vi "Main.vi"(11 "Module Admin":refnum<class "Delacor_lib_QMH_Cloneable Module Admin.lvclass">) -> ()   [LabVIEW 2019, in "Menu Module.lvlib"]
doc: "This template is based off of the Queued Message Handler design pattern and the Queued Message Handler project template that ships with LabVIEW.\n\nThe main difference is that the queue is private to this module and communication between modules is performed via Broadcast and Request events.\n\nRequest events are wrapped in public API methods and are handled in the Event Handling Loop (EHL) of this VI. Any module can register for Broadcast events sent by this module. The EHL generates messages based on user interface actions.\n\nThe Message Handling Loop (MHL) processes messages generated by the EHL, or by other messages. The messages are string values, so new messages can be added easily to the Message Cases case structure in the MHL. Each message cluster can also provide an optional value for Message Data, which is a variant that can be converted to whatever message-specific data is required.\n_____\nBased on Delacor QMH Project Template 5.0.0.82."
uses:
  Menu Module.lvlib
  <vilib>/Delacor/Delacor QMH/Libraries/Cloneable Module Admin_class/Delacor_lib_QMH_Cloneable Module Admin.lvclass
  C:/Program Files (x86)/National Instruments/LabVIEW 2019/vi.lib/Delacor/Delacor QMH/Libraries/Module Admin_class/Delacor_lib_QMH_Module Admin.lvclass
  Utility/Controls/Menu_Configuration.ctl
  Module Data--cluster.ctl
  <vilib>/Delacor/Delacor QMH/Libraries/Message Queue_class/Delacor_lib_QMH_Message Queue.lvclass/Delacor_lib_QMH_Message Queue.ctl
  <vilib>/Delacor/Delacor QMH/Libraries/Cloneable Module Admin_class/Delacor_lib_QMH_Cloneable Module Admin.lvclass/Delacor_lib_QMH_Cloneable Module Admin.ctl
  Stop Argument--cluster.ctl
  <vilib>/Delacor/Delacor QMH/Libraries/Module Admin_class/Delacor_lib_QMH_Module Admin.lvclass/Delacor_lib_QMH_Module Admin.ctl
  Init Menu Argument--cluster.ctl
  Resize the Panel Argument--cluster.ctl
  <vilib>/Utility/miscctls.llb/LVPointTypeDef.ctl
  <vilib>/Utility/miscctls.llb/LVRectTypeDef.ctl
  <vilib>/Delacor/Delacor QMH/Libraries/Message Queue_class/Delacor_lib_QMH_Enqueue Message (Single).vi
  <vilib>/Delacor/Delacor QMH/Libraries/Cloneable Module Admin_class/Delacor_lib_QMH_Get Module ID.vi
  <vilib>/Delacor/Delacor QMH/Libraries/Module Admin_class/Delacor_lib_QMH_Get External Launch.vi
  <vilib>/Utility/error.llb/Error Cluster From Error Code.vi
  <vilib>/ErrorRing/Error Ring.xnode
  <vilib>/Delacor/Delacor QMH/Libraries/Message Queue_class/Delacor_lib_QMH_Message Queue.lvclass
panel:
  in  "Select Module":i32(ring)=-1 caption="Select Module\nTo send Request to" items=["All"=-1]
  in  "Menu":T1(array[cluster])
  in  "Simulate MHL Error":bool
  in  "Simulate EHL Error":bool
  out "error out":errorcluster
  out "Status":string
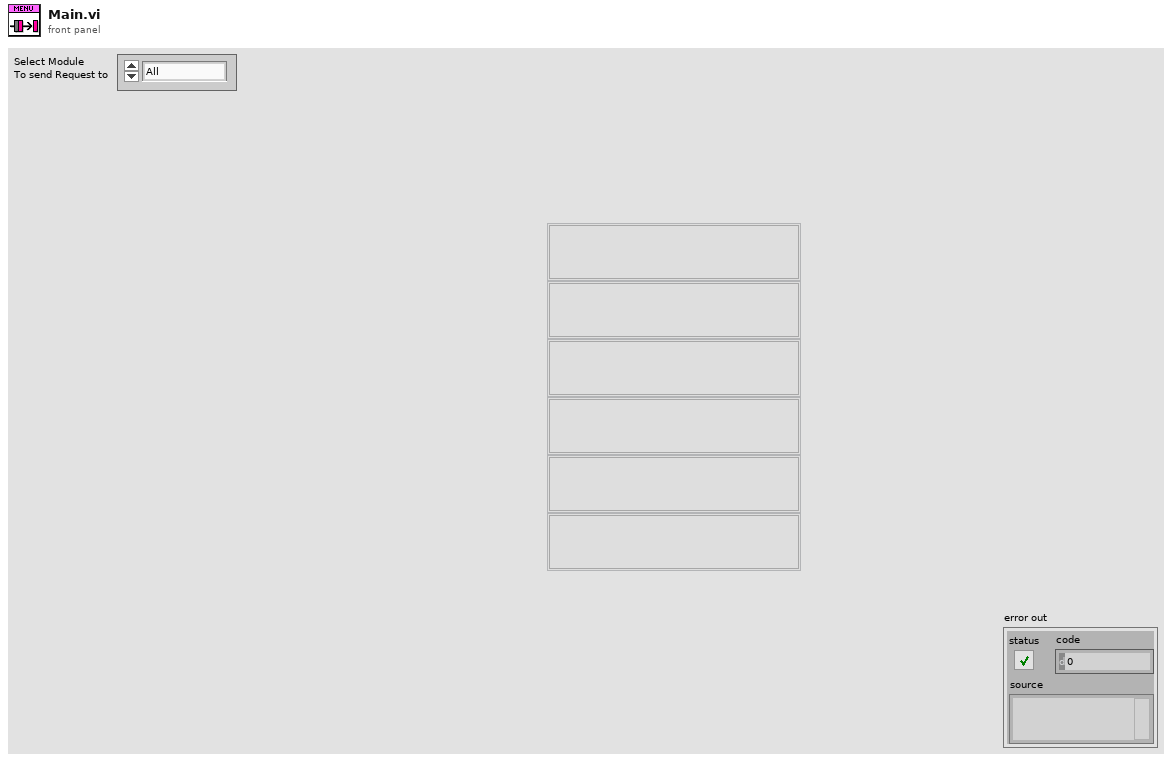
[diagram p1: front panel]
types:
  T1 = cluster{"Text ":string, "Icon":picture, "Button":bool, "Sub Menu":picture}[]
  T2 = typedef "Menu_Configuration.ctl" = cluster{"Button_Label_Color":u32, "Button_Color_On":u32, "Button_Color_Off":u32, "Panel_Color":u32, "Extend_Sub_Menu_Icon":path, "Root_Menu_Data":cluster{"Button_Icon":path, "Button_Label":string, "Sub_Menu_Data":cluster{"Button_Icon":path, "Button_Label":string, "Child_Menu_Data":cluster{"Button_Icon":path, "Button_Label":string}[]}[]}[]}
  T3 = cluster{"Text":string, "Menu_Configuration":T2, "Menu Type":enum16{"Root", "Sub", "Child"}, "Position":cluster{"Top":i16, "Left":i16}}
  T4 = typedef "Menu Module.lvlib/Request Events--cluster.ctl" = cluster{"Stop Module":refnum<user-event>, "Show Panel":refnum<user-event>, "Hide Panel":refnum<user-event>, "Show Diagram":refnum<user-event>, "Get Module Execution Status":refnum<user-event>, "Init Menu":refnum<user-event>, "Resize the Panel":refnum<user-event>}
  T5 = typedef "Menu Module.lvlib/Broadcast Events--cluster.ctl" = cluster{"Module Did Init":refnum<user-event>, "Status Updated":refnum<user-event>, "Error Reported":refnum<user-event>, "Module Did Stop":refnum<user-event>, "Update Module Execution Status":refnum<user-event>, "Button Pressed":refnum<user-event>}
  T6 = typedef "Menu Module.lvlib/Module Data--cluster.ctl" = cluster{"Status":string, "Menu_Configuration":T2, "Menu Type":enum16{"Root", "Sub", "Child"}, "Parent Name":string}
  T7 = enum32{"invalid lock state", "Not Locked", "Locked (No Password)", "Password-protected"}
  T8 = typedef "Menu Module.lvlib/Stop Argument--cluster.ctl" = cluster{"Module ID":i32, "Origin":string, "Exit via Stop Module Req?":bool, "Wait for Module to stop?":bool}
  T9 = typedef "Menu Module.lvlib/Init Menu Argument--cluster.ctl" = cluster{"Module ID":i32, "Menu_Configuration":T2, "Menu Type":enum16{"Root", "Sub", "Child"}, "Parent Name":string}
  T10 = typedef "Menu Module.lvlib/Resize the Panel Argument--cluster.ctl" = cluster{"Module ID":i32, "Boolean":bool, "Position":cluster{"Top":i16, "Left":i16}}
  T11 = typedef "LVPointTypeDef.ctl" = cluster{"Horizontal":i16, "Vertical":i16}
  T12 = enum32{"Invalid", "Standard", "Closed", "Hidden", "Minimized", "Maximized"}
  T13 = typedef "LVRectTypeDef.ctl" = cluster{"Left":i16, "Top":i16, "Right":i16, "Bottom":i16}
  T14 = typedef "LVPoint32TypeDef.ctl" = cluster{"Horizontal":i32, "Vertical":i32}
  T15 = typedef "LVPositionTypeDef.ctl" = cluster{"Left":i32, "Top":i32}
  T16 = cluster{"Text ":string, "Icon":picture, "Button":bool, "Sub Menu":picture}
  T17 = typedef "LVBoundsTypeDef.ctl" = cluster{"Width":u32, "Height":u32}
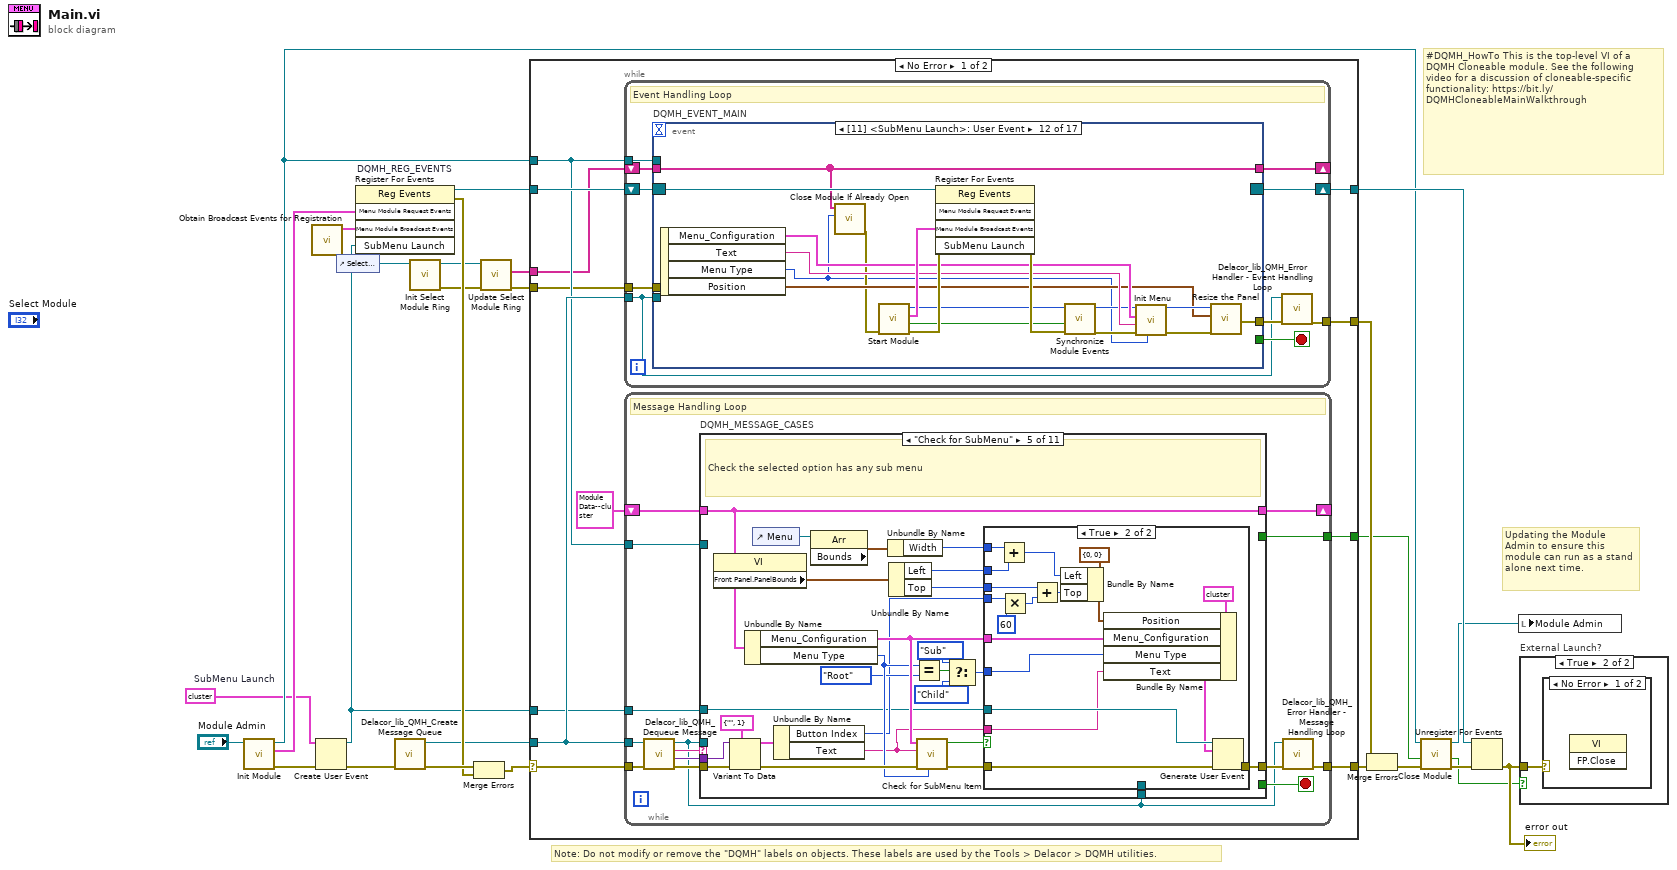
[diagram p0: block diagram]
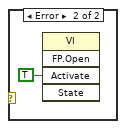
[diagram p3: hidden frame]
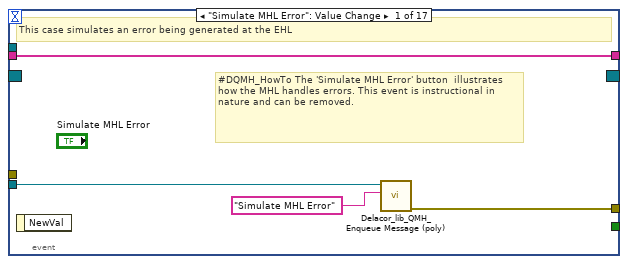
[diagram p4: hidden frame]
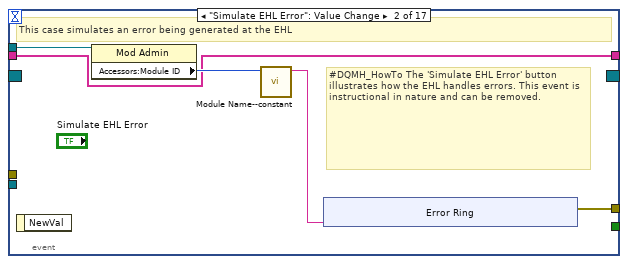
[diagram p5: hidden frame]
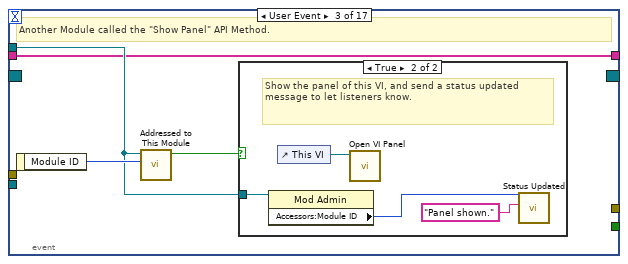
[diagram p6: hidden frame]
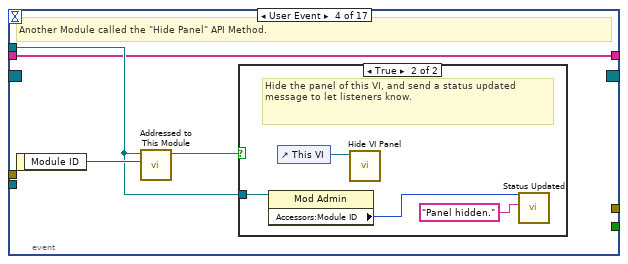
[diagram p8: hidden frame]
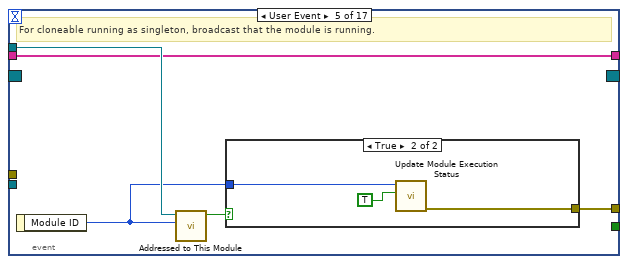
[diagram p10: hidden frame]
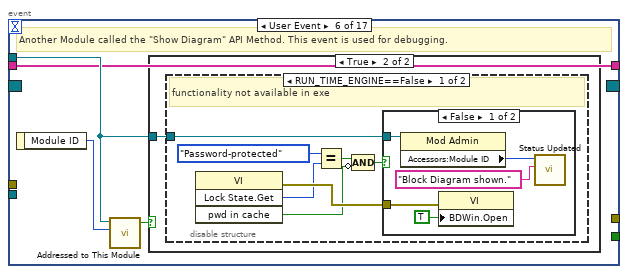
[diagram p12: hidden frame]
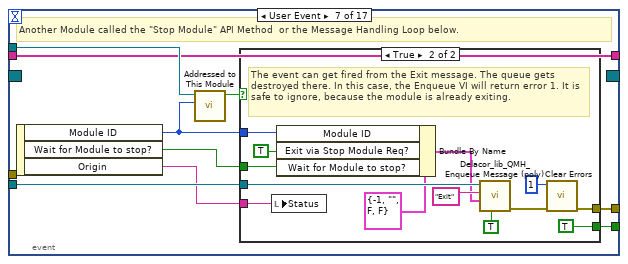
[diagram p16: hidden frame]
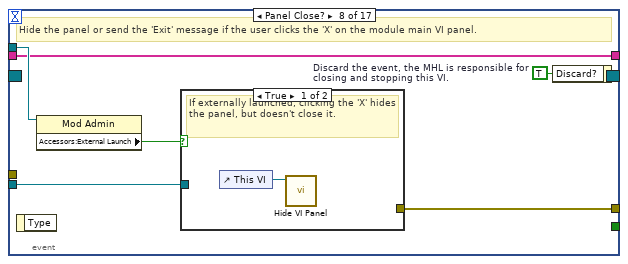
[diagram p18: hidden frame]
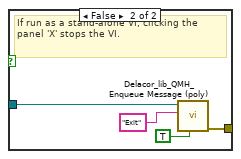
[diagram p19: hidden frame]
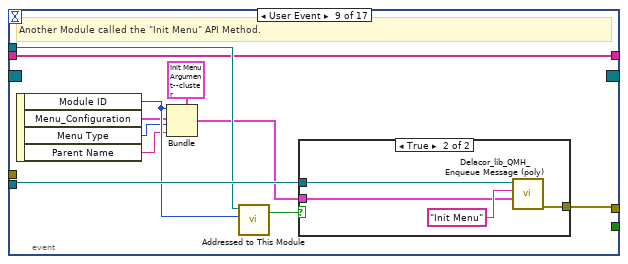
[diagram p20: hidden frame]
diagram:
  w6 = T3 {"Text"="", "Menu_Configuration"={"Button_Label_Color"=2344, "Button_Color_On"=5654, "Button_Color_Off"=2344, "Panel_Color"=2344, "Extend_Sub_Menu_Icon"=path "C:/Users/SyncSols-4/Desktop/Icon/Accept-icon.png", "Root_Menu_Data"=[{"Button_Icon"=path "C:/Users/SyncSols-4/Desktop/Icon/Accept-icon.png", "Button_Label"="Test", "Sub_Menu_Data"=[{"Button_Icon"=path "C:/Users/SyncSols-4/Desktop/Icon/floppy-icon.png", "Button_Label"="Save", "Child_Menu_Data"=[]}, {"Button_Icon"=path "C:/Users/SyncSols-4/Desktop/Icon/folder-icon1.png", "Button_Label"="Folder", "Child_Menu_Data"=[]}, {"Button_Icon"=path "C:/Users/SyncSols-4/Desktop/Icon/delete-icon.png", "Button_Label"="Delete", "Child_Menu_Data"=[{"Button_Icon"=path "C:/Users/SyncSols-4/Desktop/Icon/add-icon.png", "Button_Label"="Add"}, {"Button_Icon"=path "C:/Users/SyncSols-4/Desktop/Icon/Stop-red-icon.png", "Button_Label"="Stop"}]}]}, {"Button_Icon"=path "C:/Users/SyncSols-4/Desktop/Icon/add-key-icon.png", "Button_Label"="Key", "Sub_Menu_Data"=[]}, {"Button_Icon"=path "C:/Users/SyncSols-4/Desktop/Icon/Categories-preferences-system-icon.png", "Button_Label"="Setting", "Sub_Menu_Data"=[]}]}, "Menu Type"=enum."Root", "Position"={"Top"=0, "Left"=0}}  # SubMenu Launch
  # "#DQMH_HowTo This is the top-level VI of a DQMH Cloneable module. See the following video for a discussion of cloneable-specific functionality: https://bit.ly/DQMHCloneableMainWalkthrough"
  # "Note: Do not modify or remove the \"DQMH\" labels on objects. These labels are used by the Tools > Delacor > DQMH utilities."
  # "Updating the Module Admin to ensure this module can run as a stand alone next time."
  n1 = call "Init Module.vi"("Cloneable Module Admin in"="Module Admin") -> ("error out"=w8:errorcluster, "Menu Module Request Events"=w17:T4, "Cloneable Module Admin out"=w14:refnum<class "Delacor_lib_QMH_Cloneable Module Admin.lvclass">)  [unwired: 8 in]
  n2 = call "Obtain Broadcast Events for Registration.vi"() -> ("Menu Module Broadcast Events"=w10:T5)  [unwired: 9 in, 2 out]
  n3 = Create User Event(user event datatype=w6, error in=w8) -> (user event=w5:refnum<user-event>, error out=w7:errorcluster)
  n4 = control-ref of="Select Module"() -> (w2:refnum<vi>)
  n5 = register-events "DQMH_REG_EVENTS"(w17, w10, w5) -> (reference out=w9:refnum<event-registration>, error out=w19:errorcluster)  [unwired: 2 in]
  n6 = call <vilib>:"Delacor_lib_QMH_Create Message Queue.vi"("error in"=w7) -> ("error out"=w21:errorcluster, "Message Queue"=w16:refnum<class "Delacor_lib_QMH_Message Queue.lvclass">)  [unwired: 9 in]
  n7 = call "Init Select Module Ring.vi"("Select Module Ring Ref"=w2) -> ("error out"=w4:errorcluster)  [unwired: 8 in, 2 out]
  n8 = Merge Errors(w21, w19) -> (w20:errorcluster)
  n9 = call "Update Select Module Ring.vi"("error in (no error)"=w4, "Select Module Ring Ref"=w2) -> ("error out"=w3:errorcluster, "Active Modules (Array)"=w1:string[])  [unwired: 7 in, 1 out]
  n10 = case shown="No Error" w20 {
    selector: w20 -> [w36 w440]
    tunnel: [w38 w439] -> w24
    tunnel: [w35 w447] -> w18
    tunnel: w9 -> [w33 w447]
    tunnel: w16 -> [w32 w438]
    tunnel: [w37 _] -> w25
    tunnel: w14 -> [w31 w443]
    tunnel: [w30 _] -> w12
    tunnel: w5 -> [w29 _]
    tunnel: w3 -> [w28 _]
    tunnel: w1 -> [w27 _]
    frame No Error {
      n11 = while {
        tunnel: w32 -> [w42]
        shift-right: [w45] -> w35
        shift-left: w33 -> [w46]
        tunnel: [w47] -> w37
        tunnel: w31 -> [w43]
        shift-right: [w41] -> _
        shift-left: w27 -> [w40]
        tunnel: w28 -> [w39]
        stop <- w44 stop-if-true
        # "Event Handling Loop"
        n12 = event "DQMH_EVENT_MAIN" shown="[11] <SubMenu Launch>: User Event" {
          selector: w46 -> [_ _ _ _ _ _ _ _ _ _ _ w195 _ w209 w213 _ _]
          dyn-events: [_ _ _ _ _ _ _ _ _ _ _ _ _ w207 w213 _ _] -> w45
          timeout: _ -> [_ _ _ _ _ _ _ _ _ _ _ _ _ _ _ _ _]
          tunnel: [_ _ _ _ _ _ w110 _ _ _ _ _ _ _ _ _ _] -> w44
          tunnel: w42 -> [w51 _ _ _ _ _ w113 w130 w149 w163 w174 _ w202 _ _ w225 _]
          tunnel: [w52 w57 _ _ w85 _ w114 w133 w142 w156 w175 w183 w203 w206 w210 w224 w238] -> w48
          tunnel: w43 -> [_ w56 w66 w74 w83 w90 w112 w131 w147 w161 _ _ w201 _ _ w223 w237]
          tunnel: [w49 w53 w65 w73 w81 w89 w106 w128 w139 w154 w168 w181 w200 w205 w212 w219 w233] -> w41
          tunnel: w40 -> [w49 w53 w65 w73 w81 w89 w106 w128 w139 w154 w168 w181 w200 _ _ w219 w233]
          tunnel: w39 -> [_ _ _ _ _ _ _ _ _ _ _ _ _ _ _ _ _]
          event "Simulate MHL Error": Value Change {
            # "#DQMH_HowTo The 'Simulate MHL Error' button  illustrates how the MHL handles errors. This event is instructional in nature and can be removed."
            # "This case simulates an error being generated at the EHL"
            n13 = event-data() -> ()  [unwired: 1 in, 1 out]
            n14 = call-poly <vilib>:"Delacor_lib_QMH_Enqueue Message (poly).vi"("Message"="Simulate MHL Error", "Message Queue in"=w51) -> ("error out"=w52:errorcluster)  [unwired: 8 in, 1 out]
          }
          event "Simulate EHL Error": Value Change {
            # "#DQMH_HowTo The 'Simulate EHL Error' button  illustrates how the EHL handles errors. This event is instructional in nature and can be removed."
            # "This case simulates an error being generated at the EHL"
            n15 = event-data() -> ()  [unwired: 1 in, 1 out]
            n16 = property class="Mod Admin"(reference=w56) -> ("Accessors:Module ID"=w55:i32)  [unwired: 1 in, 2 out]
            n17 = call "Module Name--constant.vi"("Module ID"=w55) -> ("Module Name"=w54:string)  [unwired: 10 in]
            n18 = xnode "Error Ring"("parameter 0"=w54) -> ("error out"=w57:errorcluster)
          }
          event User Event {
            # "Another Module called the \"Show Panel\" API Method."
            n19 = event-data() -> ("Module ID"=w67:i32)  [unwired: 1 in]
            n20 = call "Addressed to This Module.vi"("Module ID from Argument"=w67, "Module Admin"=w66) -> ("Addressed to this instance?"=w68:bool)  [unwired: 8 in, 1 out]
            n21 = case shown="True" w68 {
              tunnel: w66 -> [_ w70]
              frame False {
              }
              frame True {
                # "Show the panel of this VI, and send a status updated message to let listeners know."
                n22 = property class="Mod Admin"(reference=w70) -> ("Accessors:Module ID"=w69:i32)  [unwired: 1 in, 2 out]
                n23 = control-ref of="This VI"() -> (w72:refnum<vi>)
                n24 = call "Open VI Panel.vi"("VI"=w72) -> ()  [unwired: 10 in, 1 out]
                n25 = call "Status Updated.vi"("Status"="Panel shown." ("format string"), "Module ID"=w69) -> ()  [unwired: 9 in, 1 out]
              }
            }
          }
          event User Event {
            # "Another Module called the \"Hide Panel\" API Method."
            n26 = event-data() -> ("Module ID"=w75:i32)  [unwired: 1 in]
            n27 = call "Addressed to This Module.vi"("Module ID from Argument"=w75, "Module Admin"=w74) -> ("Addressed to this instance?"=w76:bool)  [unwired: 8 in, 1 out]
            n28 = case shown="True" w76 {
              tunnel: w74 -> [_ w78]
              frame False {
              }
              frame True {
                # "Hide the panel of this VI, and send a status updated message to let listeners know."
                n29 = property class="Mod Admin"(reference=w78) -> ("Accessors:Module ID"=w77:i32)  [unwired: 1 in, 2 out]
                n30 = control-ref of="This VI"() -> (w80:refnum<vi>)
                n31 = call "Hide VI Panel.vi"("VI"=w80) -> ()  [unwired: 10 in, 1 out]
                n32 = call "Status Updated.vi"("Status"="Panel hidden." ("format string"), "Module ID"=w77) -> ()  [unwired: 9 in, 1 out]
              }
            }
          }
          event User Event {
            # "For cloneable running as singleton, broadcast that the module is running."
            n33 = event-data() -> ("Module ID"=w82:i32)  [unwired: 1 in]
            n34 = call "Addressed to This Module.vi"("Module ID from Argument"=w82, "Module Admin"=w83) -> ("Addressed to this instance?"=w84:bool)  [unwired: 8 in, 1 out]
            n35 = case shown="True" w84 {
              tunnel: [_ w88] -> w85
              tunnel: w82 -> [_ w87]
              frame False {
              }
              frame True {
                n36 = call "Update Module Execution Status.vi"("Running?"=TRUE, "Module ID"=w87) -> ("error out"=w88:errorcluster)  [unwired: 9 in]
              }
            }
          }
          event User Event {
            # "Another Module called the \"Show Diagram\" API Method. This event is used for debugging."
            n37 = event-data() -> ("Module ID"=w91:i32)  [unwired: 1 in]
            n38 = call "Addressed to This Module.vi"("Module ID from Argument"=w91, "Module Admin"=w90) -> ("Addressed to this instance?"=w92:bool)  [unwired: 8 in, 1 out]
            n39 = case shown="True" w92 {
              tunnel: w90 -> [_ w93]
              frame False {
              }
              frame True {
                n40 = disable-structure shown="RUN_TIME_ENGINE==False" {
                  disable-tunnel: w93 -> [w94 _]
                  frame condition #0 (active) {
                    # "functionality not available in exe"
                    n41 = invoke class="VI" method="Lock State.Get"() -> (error out=w100:errorcluster, "Get Lock State"=w99:T7, "pwd in cache"=w96:bool)  [unwired: 4 in, 1 out]
                    n42 = Equal?(x=T7."Password-protected", y=w99) -> (x = y?=w97:bool)
                    n43 = Compound Arithmetic op=AND(w97, invert w96) -> (w95:bool)
                    n44 = case shown="False" w95 {
                      tunnel: w100 -> [w105 _]
                      tunnel: w94 -> [w102 _]
                      frame False {
                        n45 = property class="Mod Admin"(reference=w102) -> ("Accessors:Module ID"=w101:i32)  [unwired: 1 in, 2 out]
                        n46 = property class="VI"(error in=w105, "BDWin.Open"=TRUE ("Block Diagram Window:Open")) -> ()  [unwired: 1 in, 2 out]
                        n47 = call "Status Updated.vi"("Status"="Block Diagram shown." ("format string"), "Module ID"=w101) -> ()  [unwired: 9 in, 1 out]
                      }
                      frame True {
                        # "Password-protected VI, and the password is not in the cache. Do not show the diagram."
                      }
                    }
                  }
                  frame condition #1 {
                  }
                }
              }
            }
          }
          event User Event {
            # "Another Module called the \"Stop Module\" API Method  or the Message Handling Loop below."
            n48 = event-data() -> ("Module ID"=w108:i32, "Wait for Module to stop?"=w109:bool, "Origin"=w107:string)  [unwired: 1 in]
            n49 = call "Addressed to This Module.vi"("Module ID from Argument"=w108, "Module Admin"=w112) -> ("Addressed to this instance?"=w111:bool)  [unwired: 8 in, 1 out]
            n50 = case shown="True" w111 {
              tunnel: [_ w126] -> w114
              tunnel: w113 -> [_ w122]
              tunnel: [_ TRUE] -> w110
              tunnel: w109 -> [_ w117]
              tunnel: w108 -> [_ w119]
              tunnel: w107 -> [_ w115]
              frame False {
              }
              frame True {
                # "The event can get fired from the Exit message. The queue gets destroyed there. In this case, the Enqueue VI will return error 1. It is safe to ignore, because the module is already exiting."
                n51 = local write "Status"(w115) -> ()
                n52 = Bundle By Name(cluster=T8 {"Module ID"=-1, "Origin"="", "Exit via Stop Module Req?"=FALSE, "Wait for Module to stop?"=FALSE} ("Stop Argument"), "Module ID"=w119, "Exit via Stop Module Req?"=TRUE, "Wait for Module to stop?"=w117) -> (w116:T8)
                n53 = call-poly <vilib>:"Delacor_lib_QMH_Enqueue Message (poly).vi"("Priority Message? (F)"=TRUE, "Message Data"=w116, "Message"="Exit", "Message Queue in"=w122) -> ("error out"=w127:errorcluster)  [unwired: 6 in, 1 out]
                n54 = call <vilib>:"Clear Errors.vi"("error in (no error)"=w127, "specific error code to clear (0: all)"=1) -> ("error out"=w126:errorcluster)  [unwired: 4 in, 1 out]
              }
            }
          }
          event Panel Close? {
            w132 = TRUE  # Discard the event, the MHL is responsible for closing and stopping this VI.
            # "Hide the panel or send the 'Exit' message if the user clicks the 'X' on the module main VI panel."
            n55 = event-data() -> ()  [unwired: 1 in, 1 out]
            n56 = property class="Mod Admin"(reference=w131) -> ("Accessors:External Launch"=w129:bool)  [unwired: 1 in, 2 out]
            n57 = case shown="True" w129 {
              tunnel: w130 -> [_ w137]
              tunnel: [_ w138] -> w133
              frame True {
                # "If externally launched, clicking the 'X' hides the panel, but doesn't close it."
                n58 = control-ref of="This VI"() -> (w134:refnum<vi>)
                n59 = call "Hide VI Panel.vi"("VI"=w134) -> ()  [unwired: 10 in, 1 out]
              }
              frame False {
                # "If run as a stand-alone VI, clicking the panel 'X' stops the VI."
                n60 = call-poly <vilib>:"Delacor_lib_QMH_Enqueue Message (poly).vi"("Priority Message? (F)"=TRUE, "Message"="Exit", "Message Queue in"=w137) -> ("error out"=w138:errorcluster)  [unwired: 7 in, 1 out]
              }
            }
            n61 = event-data("Discard?"=w132) -> ()  [unwired: 1 in, 1 out]
          }
          event User Event {
            # "Another Module called the \"Init Menu\" API Method."
            n62 = event-data() -> ("Module ID"=w144:i32, "Menu_Configuration"=w143:T2, "Menu Type"=w141:enum16{"Root", "Sub", "Child"}, "Parent Name"=w140:string)  [unwired: 1 in]
            n63 = Bundle(cluster=T9 {"Module ID"=-1, "Menu_Configuration"={"Button_Label_Color"=2344, "Button_Color_On"=5654, "Button_Color_Off"=2344, "Panel_Color"=2344, "Extend_Sub_Menu_Icon"=path "C:/Users/SyncSols-4/Desktop/Icon/Accept-icon.png", "Root_Menu_Data"=[{"Button_Icon"=path "C:/Users/SyncSols-4/Desktop/Icon/Accept-icon.png", "Button_Label"="Test", "Sub_Menu_Data"=[{"Button_Icon"=path "C:/Users/SyncSols-4/Desktop/Icon/floppy-icon.png", "Button_Label"="Save", "Child_Menu_Data"=[]}, {"Button_Icon"=path "C:/Users/SyncSols-4/Desktop/Icon/folder-icon1.png", "Button_Label"="Folder", "Child_Menu_Data"=[]}, {"Button_Icon"=path "C:/Users/SyncSols-4/Desktop/Icon/delete-icon.png", "Button_Label"="Delete", "Child_Menu_Data"=[{"Button_Icon"=path "C:/Users/SyncSols-4/Desktop/Icon/add-icon.png", "Button_Label"="Add"}, {"Button_Icon"=path "C:/Users/SyncSols-4/Desktop/Icon/Stop-red-icon.png", "Button_Label"="Stop"}]}]}, {"Button_Icon"=path "C:/Users/SyncSols-4/Desktop/Icon/add-key-icon.png", "Button_Label"="Key", "Sub_Menu_Data"=[]}, {"Button_Icon"=path "C:/Users/SyncSols-4/Desktop/Icon/Categories-preferences-system-icon.png", "Button_Label"="Setting", "Sub_Menu_Data"=[]}]}, "Menu Type"=enum."Root", "Parent Name"=""} ("Init Menu Argument"), "Module ID"=w144, "Menu_Configuration"=w143, "Menu Type"=w141, "Parent Name"=w140) -> (w145:T9)
            n64 = call "Addressed to This Module.vi"("Module ID from Argument"=w144, "Module Admin"=w147) -> ("Addressed to this instance?"=w148:bool)  [unwired: 8 in, 1 out]
            n65 = case shown="True" w148 {
              tunnel: w149 -> [_ w153]
              tunnel: w145 -> [_ w151]
              tunnel: [_ w150] -> w142
              frame False {
              }
              frame True {
                n66 = call-poly <vilib>:"Delacor_lib_QMH_Enqueue Message (poly).vi"("Message Data"=w151, "Message"="Init Menu", "Message Queue in"=w153) -> ("error out"=w150:errorcluster)  [unwired: 7 in, 1 out]
              }
            }
          }
          event User Event {
            # "Another Module called the \"Resize the Panel\" API Method."
            n67 = event-data() -> ("Module ID"=w158:i32, "Boolean"=w157:bool, "Position"=w155:cluster{"Top":i16, "Left":i16})  [unwired: 1 in]
            n68 = Bundle(cluster=T10 {"Module ID"=-1, "Boolean"=FALSE, "Position"={"Top"=100, "Left"=100}} ("Resize the Panel Argument"), "Module ID"=w158, "Boolean"=w157, "Position"=w155) -> (w159:T10)
            n69 = call "Addressed to This Module.vi"("Module ID from Argument"=w158, "Module Admin"=w161) -> ("Addressed to this instance?"=w162:bool)  [unwired: 8 in, 1 out]
            n70 = case shown="True" w162 {
              tunnel: w163 -> [_ w167]
              tunnel: w159 -> [_ w165]
              tunnel: [_ w164] -> w156
              frame False {
              }
              frame True {
                n71 = call-poly <vilib>:"Delacor_lib_QMH_Enqueue Message (poly).vi"("Message Data"=w165, "Message"="Resize the Panel", "Message Queue in"=w167) -> ("error out"=w164:errorcluster)  [unwired: 7 in, 1 out]
              }
            }
          }
          event "Menu": Mouse Down {
            n72 = event-data() -> ("Coords"=w179:T14)  [unwired: 1 in]
            n73 = property on="Menu" class="Arr"() -> ("Position"=w178:T15)  [unwired: 2 in, 2 out]
            n74 = call "Find Mouse Down Option.vi"("Menu Position"=w178, "Mouse DownCoords"=w179) -> ("Button Index"=w171:u32)  [unwired: 8 in, 1 out]
            n75 = Index Array(array="Menu", index=w171) -> (element=w176:T16)
            n76 = Unbundle By Name(w176) -> ("Text"=w172:string)
            n77 = Bundle By Name(cluster=cluster{"Text":string, "Button Index":u32} {"Text"="", "Button Index"=1}, "Text"=w172, "Button Index"=w171) -> (w170:cluster{"Text":string, "Button Index":u32})
            n78 = call-poly <vilib>:"Delacor_lib_QMH_Enqueue Message (poly).vi"("Message Data"=w170, "Message"="Check for SubMenu", "Message Queue in"=w174) -> ("error out"=w175:errorcluster)  [unwired: 7 in, 1 out]
          }
          event User Event {
            n79 = event-data() -> ("Menu_Configuration"=w188:T2, "Text"=w187:string, "Menu Type"=w180:enum16{"Root", "Sub", "Child"}, "Position"=w184:cluster{"Top":i16, "Left":i16})  [unwired: 1 in]
            n80 = call "Close Module If Already Open.vi"("Menu Type"=w180, "Module List"=w181) -> ("error out"=w182:errorcluster)  [unwired: 9 in]
            n81 = call "Start Module.vi"("error in (no error)"=w182) -> ("error out"=w193:errorcluster, "Wait for Event Sync?"=w190:bool, "Menu Module Broadcast Events"=w194:T5, "Module ID"=w191:i32)  [unwired: 7 in]
            n82 = register-events(reference=w195, error in=w193, w194) -> (error out=w192:errorcluster)  [unwired: 2 in, 1 out]
            n83 = call "Synchronize Module Events.vi"("error in (no error)"=w192, "Wait for Event Sync?"=w190, "Module ID"=w191) -> ("error out"=w189:errorcluster, "Module ID (dup)"=w186:i32)  [unwired: 7 in]
            n84 = call "Init Menu.vi"("Menu Type"=w180, "error in (no error)"=w189, "Parent Name"=w187, "Menu_Configuration"=w188, "Module ID"=w186) -> ("error out"=w185:errorcluster)  [unwired: 6 in]
            n85 = call "Resize the Panel.vi"("error in (no error)"=w185, "Position"=w184, "Module ID"=w186) -> ("error out"=w183:errorcluster)  [unwired: 8 in]
          }
          event User Event {
            n86 = event-data() -> ()  [unwired: 1 in, 1 out]
            n87 = property class="Mod Admin"(reference=w201) -> ("Accessors:Module ID"=w198:i32)  [unwired: 1 in, 2 out]
            n88 = Number To Decimal String(number=w198) -> (decimal integer string=w199:string)  [unwired: 1 in]
            n89 = Search 1D Array(1D array=w200, element=w199) -> (index of element=w197:i32)  [unwired: 1 in]
            n90 = Equal To 0?(x=w197) -> ()  [unwired: 1 out]
            n91 = call-poly <vilib>:"Delacor_lib_QMH_Enqueue Message (poly).vi"("Message"="Exit", "Message Queue in"=w202) -> ("error out"=w203:errorcluster)  [unwired: 8 in, 1 out]
          }
          event User Event {
            n92 = event-data() -> ()  [unwired: 1 in, 2 out]
            n93 = call "Obtain Broadcast Events for Registration.vi"() -> ("error out"=w206:errorcluster, "Menu Module Broadcast Events"=w208:T5)  [unwired: 9 in, 1 out]
            n94 = register-events "Reg Event"(reference=w209, w208) -> (reference out=w207:refnum<event-registration>)  [unwired: 3 in, 1 out]
            n95 = control-ref of="Select Module"() -> (w204:refnum<vi>)
            n96 = call "Update Select Module Ring.vi"("error in (no error)"=w206, "Select Module Ring Ref"=w204) -> ("Active Modules (Array)"=w205:string[])  [unwired: 7 in, 2 out]
          }
          event User Event {
            n97 = event-data() -> ()  [unwired: 1 in, 2 out]
            n98 = control-ref of="Select Module"() -> (w211:refnum<vi>)
            n99 = call "Update Select Module Ring.vi"("Select Module Ring Ref"=w211) -> ("error out"=w210:errorcluster, "Active Modules (Array)"=w212:string[])  [unwired: 8 in, 1 out]
          }
          event Mouse Leave {
            n100 = event-data() -> ()  [unwired: 1 in, 1 out]
            n101 = property class="Mod Admin"(reference=w223) -> ("Accessors:Module ID"=w220:i32)  [unwired: 1 in, 2 out]
            n102 = Number To Decimal String(number=w220) -> (decimal integer string=w222:string)  [unwired: 1 in]
            n103 = Search 1D Array(1D array=w219, element=w222) -> (index of element=w216:i32)  [unwired: 1 in]
            n104 = Array Size(array=w219) -> (size(s)=w218:i32)
            n105 = Decrement(x=w218) -> (x-1=w217:i32)
            n106 = Greater?(x=w217, y=w216) -> (0:w214:bool)
            n107 = Equal To 0?(x=w216) -> (x = 0?=w221:bool)
            n108 = Or(x=w214, y=w221) -> (x .or. y?=w215:bool)
            n109 = case "Last Module Mouse Leave" shown="False" w215 {
              tunnel: w225 -> [w227 _]
              tunnel: [w226 _] -> w224
              frame False {
                n110 = call-poly <vilib>:"Delacor_lib_QMH_Enqueue Message (poly).vi"("Message"="Exit", "Message Queue in"=w227) -> ("error out"=w226:errorcluster)  [unwired: 8 in, 1 out]
              }
              frame True {
              }
            }
          }
          event "Menu": Mouse Move {
            n111 = event-data() -> ()  [unwired: 1 in, 1 out]
            n112 = property class="Mod Admin"(reference=w237) -> ("Accessors:Module ID"=w235:i32)  [unwired: 1 in, 2 out]
            n113 = Decimal String To Number(string=w233) -> (number=w236:i32[])  [unwired: 2 in, 1 out]
            n114 = Array Size(array=w233) -> (size(s)=w231:i32)
            n115 = Search 1D Array(1D array=w236, element=w235) -> (index of element=w234:i32)  [unwired: 1 in]
            n116 = Increment(x=w234) -> (x+1=w232:i32)
            n117 = Equal?(x=w231, y=w232) -> ()  [unwired: 1 out]
            n118 = Increment(x=w235) -> (x+1=w230:i32)
            n119 = case shown="False" TRUE {
              tunnel: [w240 _] -> w238
              tunnel: w230 -> [w239 _]
              frame False {
                n120 = call "Stop Module.vi"("Module ID"=w239) -> ("error out"=w240:errorcluster)  [unwired: 10 in]
              }
              frame True {
              }
            }
          }
        }
        n121 = call-dynamic "Delacor_lib_QMH_Error Handler - Event Handling Loop.vi"("error in"=w48, "Message Queue in"=w42) -> ("dup error in"=w47:errorcluster)  [unwired: 8 in, 1 out]
      }
      n122 = while {
        tunnel: w32 -> [w245]
        shift-right: [w249] -> _
        shift-left: T6 {"Status"="", "Menu_Configuration"={"Button_Label_Color"=2344, "Button_Color_On"=5654, "Button_Color_Off"=2344, "Panel_Color"=2344, "Extend_Sub_Menu_Icon"=path "C:/Users/SyncSols-4/Desktop/Icon/Accept-icon.png", "Root_Menu_Data"=[{"Button_Icon"=path "C:/Users/SyncSols-4/Desktop/Icon/Accept-icon.png", "Button_Label"="Test", "Sub_Menu_Data"=[{"Button_Icon"=path "C:/Users/SyncSols-4/Desktop/Icon/floppy-icon.png", "Button_Label"="Save", "Child_Menu_Data"=[]}, {"Button_Icon"=path "C:/Users/SyncSols-4/Desktop/Icon/folder-icon1.png", "Button_Label"="Folder", "Child_Menu_Data"=[]}, {"Button_Icon"=path "C:/Users/SyncSols-4/Desktop/Icon/delete-icon.png", "Button_Label"="Delete", "Child_Menu_Data"=[{"Button_Icon"=path "C:/Users/SyncSols-4/Desktop/Icon/add-icon.png", "Button_Label"="Add"}, {"Button_Icon"=path "C:/Users/SyncSols-4/Desktop/Icon/Stop-red-icon.png", "Button_Label"="Stop"}]}]}, {"Button_Icon"=path "C:/Users/SyncSols-4/Desktop/Icon/add-key-icon.png", "Button_Label"="Key", "Sub_Menu_Data"=[]}, {"Button_Icon"=path "C:/Users/SyncSols-4/Desktop/Icon/Categories-preferences-system-icon.png", "Button_Label"="Setting", "Sub_Menu_Data"=[]}]}, "Menu Type"=enum."Root", "Parent Name"=""} ("Data Cluster") -> [w250]
        tunnel: w36 -> [w253]
        tunnel: [w251] -> w38
        tunnel: w31 -> [w244]
        tunnel: [w243] -> w30
        tunnel: w29 -> [w241]
        stop <- w248 stop-if-true
        # "Message Handling Loop"
        n123 = call-dynamic "Delacor_lib_QMH_Dequeue Message.vi"("error in"=w253, "Message Queue in"=w245) -> ("error out"=w252:errorcluster, "Message Data"=w246:variant, "Message"=w247:string, "Message Queue out"=w242:refnum<class "Delacor_lib_QMH_Message Queue.lvclass">)  [unwired: 6 in]
        n124 = case "DQMH_MESSAGE_CASES" shown="\"Check for SubMenu\"" w247 {
          selector: w247 -> [_ _ _ _ _ _ _ _ _ _ w425]
          tunnel: w242 -> [_ _ _ _ _ _ _ w376 _ w415 _]
          tunnel: w252 -> [w273 w277 w295 w317 w342 w371 w373 w385 w398 w421 w427]
          tunnel: [w271 w277 w285 w315 w337 w370 w373 w381 w397 w418 w428] -> w254
          tunnel: w250 -> [w264 w276 w294 w316 w340 w369 w372 w380 w395 w414 w426]
          tunnel: [w263 w276 w281 w316 w340 w369 w372 w380 w395 w414 w426] -> w249
          tunnel: [_ _ _ _ _ _ _ _ _ w413 _] -> w248
          tunnel: w246 -> [_ _ w293 w314 w343 _ _ w379 _ w411 _]
          tunnel: w244 -> [w258 _ _ _ _ _ _ w378 w393 w407 w423]
          tunnel: [_ _ _ _ _ _ _ _ _ w409 _] -> w243
          tunnel: w242 -> [_ _ _ _ w336 _ _ _ _ _ _]
          tunnel: w241 -> [_ _ _ _ w318 _ _ _ _ _ _]
          frame "Initialize" {
            w255 = "Initial Message" ("Initial Message")
            # "#CodeNeeded - Initialize the appearance of the front panel."
            # "#CodeNeeded - Initialize your state data here."
            # "Initialize - Any operation that needs to be done before the module can receive messages. Synchronize Caller Events.vi will inform Start Module.vi that the module has launched and is ready to receive messages. Module Did Init.vi will broadcast that the module initialized."
            n125 = call "Synchronize Caller Events.vi"("error in (no error)"=w273, "Module Admin"=w258) -> ("error out"=w272:errorcluster, "Module Admin out"=w257:refnum<class "Delacor_lib_QMH_Cloneable Module Admin.lvclass">)  [unwired: 8 in]
            n126 = property class="Mod Admin"(reference=w257) -> ("Accessors:Module ID"=w260:i32, "Accessors:External Launch"=w259:bool)  [unwired: 1 in, 2 out]
            n127 = call "Module Name--constant.vi"("Module ID"=w260) -> ("Module Name"=w268:string)  [unwired: 10 in]
            n128 = property class="VI"("Front Panel.Title"=w268) -> (reference out=w270:refnum<vi>, error out=w275:errorcluster)  [unwired: 2 in]
            n129 = Select(t=T12."Hidden" ("State"), s=w259, f=T12."Standard" ("State")) -> (s? t:f=w265:T12)
            n130 = invoke class="VI" method="FP.Open"(reference=w270, error in=w275, "State"=w265) -> (reference out=w269:refnum<vi>, error out=w274:errorcluster)  [unwired: 2 in, 3 out]
            n131 = call "Module Name--constant.vi"("Module ID"=w260) -> ("Module Name"=w261:string)  [unwired: 10 in]
            n132 = Bundle By Name(cluster=w264, "Status"=w255) -> (w263:T6)
            n133 = invoke class="VI" method="FP.Center"(reference=w269, error in=w274) -> ()  [unwired: 1 in, 3 out]
            n134 = property on="Pane" class="Pane"("Origin"=T11 {"Horizontal"=0, "Vertical"=0}) -> ()  [unwired: 2 in, 2 out]
            n135 = call "Module Did Init.vi"("error in (no error)"=w272, "Initialized?"=TRUE, "Origin"=w261, "Module ID"=w260) -> ("error out"=w271:errorcluster)  [unwired: 7 in]
            "Status" <- w255
          }
          frame "--- Module Specific ---" {
            # "Separator -- The following cases handle messages specific to this Module."
          }
          frame "Init Menu" {
            # "This Event Initialize the Menu Items and change the apperance of the menu"
            n136 = Variant To Data(error in=w295, type=T9 {"Module ID"=-1, "Menu_Configuration"={"Button_Label_Color"=2344, "Button_Color_On"=5654, "Button_Color_Off"=2344, "Panel_Color"=2344, "Extend_Sub_Menu_Icon"=path "C:/Users/SyncSols-4/Desktop/Icon/Accept-icon.png", "Root_Menu_Data"=[{"Button_Icon"=path "C:/Users/SyncSols-4/Desktop/Icon/Accept-icon.png", "Button_Label"="Test", "Sub_Menu_Data"=[{"Button_Icon"=path "C:/Users/SyncSols-4/Desktop/Icon/floppy-icon.png", "Button_Label"="Save", "Child_Menu_Data"=[]}, {"Button_Icon"=path "C:/Users/SyncSols-4/Desktop/Icon/folder-icon1.png", "Button_Label"="Folder", "Child_Menu_Data"=[]}, {"Button_Icon"=path "C:/Users/SyncSols-4/Desktop/Icon/delete-icon.png", "Button_Label"="Delete", "Child_Menu_Data"=[{"Button_Icon"=path "C:/Users/SyncSols-4/Desktop/Icon/add-icon.png", "Button_Label"="Add"}, {"Button_Icon"=path "C:/Users/SyncSols-4/Desktop/Icon/Stop-red-icon.png", "Button_Label"="Stop"}]}]}, {"Button_Icon"=path "C:/Users/SyncSols-4/Desktop/Icon/add-key-icon.png", "Button_Label"="Key", "Sub_Menu_Data"=[]}, {"Button_Icon"=path "C:/Users/SyncSols-4/Desktop/Icon/Categories-preferences-system-icon.png", "Button_Label"="Setting", "Sub_Menu_Data"=[]}]}, "Menu Type"=enum."Root", "Parent Name"=""} ("Init Menu Argument"), Variant=w293) -> (data=w291:T9, error out=w286:errorcluster)
            n137 = Unbundle By Name(w291) -> ("Menu_Configuration"=w280:T2, "Menu_Configuration.Button_Color_On"=w289:u32, "Menu_Configuration.Button_Label_Color"=w288:u32, "Menu_Configuration.Panel_Color"=w283:u32, "Menu_Configuration.Button_Color_Off"=w287:u32, "Parent Name"=w279:string, "Menu Type"=w278:enum16{"Root", "Sub", "Child"})
            n138 = control-ref of="This VI"() -> (w282:refnum<vi>)
            n139 = control-ref of="Menu"() -> (w284:refnum<vi>)
            n140 = call "Change_Aperence_of_the_Menu_Items.vi"("VI Ref"=w282, "Button_Color_Off"=w287, "Button_Color_On"=w289, "error in"=w286, "Panel_Color"=w283, "Button_Label_Color"=w288, "Menu"=w284) -> ("error out"=w290:errorcluster)  [unwired: 4 in]
            n141 = call "Update_Menu_Items.vi"("Menu Type"=w278, "Menu"=w284, "error in"=w290, "Parent Menu Name"=w279, "Menu_Configuration"=w280) -> ("error out"=w285:errorcluster)  [unwired: 6 in]
            n142 = Bundle By Name(cluster=w294, "Menu_Configuration"=w280, "Parent Name"=w279, "Menu Type"=w278) -> (w281:T6)
          }
          frame "Resize the Panel" {
            # "Resize the Front Panel based on the Menu Bounds"
            n143 = control-ref of="Menu"() -> (w312:refnum<vi>)
            n144 = Variant To Data(error in=w317, type=T10 {"Module ID"=-1, "Boolean"=FALSE, "Position"={"Top"=100, "Left"=100}} ("Resize the Panel Argument"), Variant=w314) -> (data=w300:T10, error out=w315:errorcluster)
            n145 = property class="Arr"(reference=w312) -> ("Bounds"=w306:T17)  [unwired: 1 in, 2 out]
            n146 = Unbundle By Name(w306) -> ("Width"=w305:u32, "Height"=w304:u32)
            n147 = Unbundle By Name(w300) -> ("Position.Top"=w298:i16, "Position.Left"=w296:i16)
            n148 = Add(x=w304, y=w298) -> (x+y=w299:u32)
            n149 = Add(x=w296, y=w305) -> (x+y=w297:u32)
            n150 = invoke class="VI" method="FP.Open"("Activate"=TRUE ("Activate?"), "State"=T12."Hidden") -> (reference out=w310:refnum<vi>, error out=w309:errorcluster)  [unwired: 3 in, 3 out]
            n151 = Bundle By Name(cluster=T13 {"Left"=100, "Top"=100, "Right"=0, "Bottom"=0} ("Front Panel Window:Panel Bounds"), "Right"=w297, "Bottom"=w299, "Top"=w298, "Left"=w296) -> (w307:T13)
            n152 = property class="VI"(reference=w310, error in=w309, "Front Panel.PanelBounds"=w307) -> (reference out=w302:refnum<vi>)  [unwired: 1 out]
            n153 = property class="VI"(reference=w302, "FP.State"=T12."Standard" ("Front Panel Window:State")) -> ()  [unwired: 1 in, 2 out]
          }
          frame "Check for SubMenu" {
            # "Check the selected option has any sub menu"
            n154 = property class="VI"() -> ("Front Panel.PanelBounds"=w322:T13)  [unwired: 2 in, 2 out]
            n155 = Variant To Data(error in=w342, type=cluster{"Text":string, "Button Index":u32} {"Text"="", "Button Index"=1}, Variant=w343) -> (data=w325:cluster{"Text":string, "Button Index":u32}, error out=w341:errorcluster)
            n156 = Unbundle By Name(w340) -> ("Menu_Configuration"=w335:T2, "Menu Type"=w334:enum16{"Root", "Sub", "Child"})
            n157 = control-ref of="Menu"() -> (w328:refnum<vi>)
            n158 = Unbundle By Name(w325) -> ("Button Index"=w323:u32, "Text"=w324:string)
            n159 = property class="Arr"(reference=w328) -> ("Bounds"=w327:T17)  [unwired: 1 in, 2 out]
            n160 = Unbundle By Name(w327) -> ("Width"=w326:u32)
            n161 = Unbundle By Name(w322) -> ("Left"=w321:i16, "Top"=w320:i16)
            n162 = Equal?(x=w334, y=enum16{"Root", "Sub", "Child"}."Root") -> (x = y?=w332:bool)
            n163 = call "Check for SubMenu Item.vi"("Menu Type"=w334, "error in"=w341, "Selected Option"=w324, "Menu_Configuration"=w335) -> ("error out"=w338:errorcluster, "Sub Menu Present?"=w339:bool)  [unwired: 6 in]
            n164 = Select(t=enum16{"Root", "Sub", "Child"}."Sub" ("y"), s=w332, f=enum16{"Root", "Sub", "Child"}."Child" ("y")) -> (s? t:f=w329:enum16{"Root", "Sub", "Child"})
            n165 = case shown="True" w339 {
              tunnel: w338 -> [w349 w359]
              tunnel: [w347 w358] -> w337
              tunnel: w324 -> [w346 w351]
              tunnel: w336 -> [w345 _]
              tunnel: w335 -> [_ w353]
              tunnel: w329 -> [_ w352]
              tunnel: w326 -> [_ w367]
              tunnel: w323 -> [_ w366]
              tunnel: w321 -> [_ w362]
              tunnel: w320 -> [_ w360]
              tunnel: w318 -> [_ w357]
              frame False {
                n166 = call "Button Pressed.vi"("error in (no error)"=w349, "selected Option"=w346, "Module ID"=-1) -> ("error out"=w348:errorcluster)  [unwired: 8 in]
                n167 = call-poly <vilib>:"Delacor_lib_QMH_Enqueue Message (poly).vi"("error in"=w348, "Message"="Exit", "Message Queue in"=w345) -> ("error out"=w347:errorcluster)  [unwired: 7 in, 1 out]
              }
              frame True {
                n168 = Add(x=w367, y=w362) -> (x+y=w363:u32)
                n169 = Multiply(x=w366, y=60) -> (x*y=w364:u32)
                n170 = Add(x=w360, y=w364) -> (x+y=w361:u32)
                n171 = Bundle By Name(cluster=cluster{"Top":i16, "Left":i16} {"Top"=0, "Left"=0} ("Position"), "Left"=w363, "Top"=w361) -> (w354:cluster{"Top":i16, "Left":i16})
                n172 = Bundle By Name(cluster=T3 {"Text"="", "Menu_Configuration"={"Button_Label_Color"=2344, "Button_Color_On"=5654, "Button_Color_Off"=2344, "Panel_Color"=2344, "Extend_Sub_Menu_Icon"=path "C:/Users/SyncSols-4/Desktop/Icon/Accept-icon.png", "Root_Menu_Data"=[{"Button_Icon"=path "C:/Users/SyncSols-4/Desktop/Icon/Accept-icon.png", "Button_Label"="Test", "Sub_Menu_Data"=[{"Button_Icon"=path "C:/Users/SyncSols-4/Desktop/Icon/floppy-icon.png", "Button_Label"="Save", "Child_Menu_Data"=[]}, {"Button_Icon"=path "C:/Users/SyncSols-4/Desktop/Icon/folder-icon1.png", "Button_Label"="Folder", "Child_Menu_Data"=[]}, {"Button_Icon"=path "C:/Users/SyncSols-4/Desktop/Icon/delete-icon.png", "Button_Label"="Delete", "Child_Menu_Data"=[{"Button_Icon"=path "C:/Users/SyncSols-4/Desktop/Icon/add-icon.png", "Button_Label"="Add"}, {"Button_Icon"=path "C:/Users/SyncSols-4/Desktop/Icon/Stop-red-icon.png", "Button_Label"="Stop"}]}]}, {"Button_Icon"=path "C:/Users/SyncSols-4/Desktop/Icon/add-key-icon.png", "Button_Label"="Key", "Sub_Menu_Data"=[]}, {"Button_Icon"=path "C:/Users/SyncSols-4/Desktop/Icon/Categories-preferences-system-icon.png", "Button_Label"="Setting", "Sub_Menu_Data"=[]}]}, "Menu Type"=enum."Root", "Position"={"Top"=0, "Left"=0}} ("SubMenu Launch"), "Position"=w354, "Menu_Configuration"=w353, "Menu Type"=w352, "Text"=w351) -> (w355:T3)
                n173 = Generate User Event(user event=w357, event data cluster=w355, error in=w359) -> (error out=w358:errorcluster)  [unwired: 1 in, 1 out]
              }
            }
          }
          frame "---Copy This Frame---" {
            # "Duplicate this frame when creating new messages.  Change this comment in the duplicated frame to describe this message."
            n174 = Merge Errors(w371) -> (w370:errorcluster)
          }
          frame "--- Exit and Error Handling---" {
            # "Separator - the following cases handle errors and exit messages."
          }
          frame "Error" {
            # "#CodeRecommended - If you ever change the name of this \"Error\" message, you'll need to update the name in the Check Loop Error.vi as well."
            # "#CodeRecommended - If the module is running in standalone mode (External Launch = FALSE), this code will pop up an error dialog and call the 'Exit' message if an error occurs. Add more fine-grained error handling here."
            # "Error - Check the error message data and respond accordingly. This message is sent by the \"Error Handler\" VIs at the end of each loop in this application."
            n175 = property class="Mod Admin"(reference=w378) -> ("Accessors:External Launch"=w377:bool, "Accessors:Module ID"=w374:i32)  [unwired: 1 in, 2 out]
            n176 = Variant To Data(error in=w385, type=errorcluster {"status"=FALSE, "code"=0, "source"=""} ("error constant"), Variant=w379) -> (data=w386:errorcluster, error out=w383:errorcluster)
            n177 = call "Module Name--constant.vi"("Module ID"=w374) -> ("Module Name"=w375:string)  [unwired: 10 in]
            n178 = call "Error Reported.vi"("Additional Information"=w375, "Error"=w386, "Module ID"=w374) -> ()  [unwired: 8 in, 1 out]
            n179 = case shown="False" w377 {
              tunnel: [w391 _] -> w382
              tunnel: w376 -> [w389 _]
              tunnel: w386 -> [w390 _]
              frame False {
                # "If the module is running standalone, then pop up an error dialog and call the \"Exit\" message."
                n180 = call <vilib>:"Simple Error Handler.vi"("error in (no error)"=w390) -> ()  [unwired: 4 in, 5 out]
                n181 = call-poly <vilib>:"Delacor_lib_QMH_Enqueue Message (poly).vi"("Priority Message? (F)"=TRUE, "Message"="Exit", "Message Queue in"=w389) -> ("error out"=w391:errorcluster)  [unwired: 7 in, 1 out]
              }
              frame True {
                # "If the module was launched externally, calling the Error Reported broadcast VI is the only action performed by the \"Error\" message. The module's caller can then process the error appropriately."
              }
            }
            n182 = Merge Errors(w383, w382) -> (w381:errorcluster)
            n183 = local write "error out"(w381) -> ()
          }
          frame "Simulate MHL Error" {
            # "#DQMH_HowTo The 'Simulate MHL Error' button  illustrates how the MHL handles errors. This event is instructional in nature and can be removed."
            # "Simulate an error occurring at the MHL"
            n184 = property class="Mod Admin"(reference=w393) -> ("Accessors:Module ID"=w394:i32)  [unwired: 1 in, 2 out]
            n185 = call "Module Name--constant.vi"("Module ID"=w394) -> ("Module Name"=w392:string)  [unwired: 10 in]
            n186 = xnode "Error Ring"("parameter 0"=w392) -> ("error out"=w396:errorcluster)
            n187 = Merge Errors(w398, w396) -> (w397:errorcluster)
          }
          frame "Exit" {
            w412 = 91  # 91: not all Exit messages will have an argument
            w413 = TRUE  # Stop the VI
            # "Release the message queue reference"
            # "#CodeNeeded - Add any required cleanup code here."
            # "Exit - Exit the application."
            n188 = Variant To Data(error in=w421, type=T8 {"Module ID"=-1, "Origin"="", "Exit via Stop Module Req?"=FALSE, "Wait for Module to stop?"=FALSE} ("Stop Argument"), Variant=w411) -> (data=w408:T8, error out=w416:errorcluster)
            n189 = call <vilib>:"Clear Errors.vi"("error in (no error)"=w416, "specific error code to clear (0: all)"=w412) -> ("error out"=w420:errorcluster)  [unwired: 4 in, 1 out]
            n190 = control-ref of="This VI"() -> (w406:refnum<vi>)
            n191 = call-dynamic "Delacor_lib_QMH_Release Message Queue.vi"("error in"=w420, "Message Queue"=w415) -> ("error out"=w419:errorcluster)  [unwired: 9 in]
            n192 = call "Handle Exit.vi"("Stop Argument"=w408, "Module Admin in"=w407, "VI reference"=w406) -> ("error out"=w417:errorcluster, "Wait for Stop?"=w409:bool)  [unwired: 7 in]
            n193 = Merge Errors(w419, w417) -> (w418:errorcluster)
          }
          frame Default {
            # "'Default' case only runs if there is a message that isn't defined in any of the other cases.  Output a programming error."
            n194 = property class="Mod Admin"(reference=w423) -> ("Accessors:Module ID"=w422:i32)  [unwired: 1 in, 2 out]
            n195 = call "Module Name--constant.vi"("Module ID"=w422) -> ("Module Name"=w424:string)  [unwired: 10 in]
            n196 = xnode "Error Ring"("parameter 0"=w425, "parameter 1"=w424) -> ("error out"=w429:errorcluster)
            n197 = Merge Errors(w427, w429) -> (w428:errorcluster)
          }
        }
        n198 = call-dynamic "Delacor_lib_QMH_Error Handler - Message Handling Loop.vi"("error in"=w254, "Message Queue in"=w242) -> ("dup error in"=w251:errorcluster)  [unwired: 8 in, 1 out]
      }
    }
    frame Error {
      n199 = call "Synchronize Caller Events.vi"("Module Admin"=w443) -> ("Module Admin out"=w442:refnum<class "Delacor_lib_QMH_Cloneable Module Admin.lvclass">)  [unwired: 9 in, 1 out]
      n200 = property class="Mod Admin"(reference=w442) -> ("Accessors:Module ID"=w441:i32)  [unwired: 1 in, 2 out]
      n201 = call-dynamic "Delacor_lib_QMH_Release Message Queue.vi"("error in"=w440, "Message Queue"=w438) -> ("error out"=w439:errorcluster)  [unwired: 9 in]
      n202 = call "Module Name--constant.vi"("Module ID"=w441) -> ("Module Name"=w446:string)  [unwired: 10 in]
      n203 = Format Into String(format string="An error occurred during initialization. %s is no longer running.", w446) -> (resulting string=w444:string)  [unwired: 2 in, 1 out]
      n204 = call "Error Reported.vi"("Additional Information"=w444, "Error"=w439, "Module ID"=w441) -> ()  [unwired: 8 in, 1 out]
    }
  }
  n205 = Merge Errors(w25, w24) -> (w26:errorcluster)
  n206 = call "Close Module.vi"("error in"=w26, "Wait for stop?"=w12, "Module Admin in"=w14) -> ("error out"=w23:errorcluster, "External Launch"=w11:bool, "Module Admin out"=w13:refnum<class "Delacor_lib_QMH_Cloneable Module Admin.lvclass">)  [unwired: 6 in]
  n207 = Unregister For Events(event registration refnum=w18, error in=w23) -> (error out=w22:errorcluster)
  "error out" <- w22
  n208 = local write "Module Admin"(w13) -> ()
  n209 = case "External Launch?" shown="True" w11 {
    tunnel: w22 -> [_ w448]
    frame False {
    }
    frame True {
      n210 = case shown="No Error" w448 {
        frame No Error {
          n211 = invoke class="VI" method="FP.Close"() -> ()  [unwired: 3 in, 3 out]
        }
        frame Error {
          n212 = invoke class="VI" method="FP.Open"("Activate"=TRUE ("Activate?")) -> ()  [unwired: 4 in, 5 out]
        }
      }
    }
  }
